vi "Shift Rev.vi"(10 "iterator":refnum<data-value>, 11 "INode in":refnum<class "INode.lvclass">) -> (3 "INode out":refnum<class "INode.lvclass">)   [LabVIEW 2023, in "d20.lvlib" / "INode.lvclass"]
uses:
  INode.lvclass
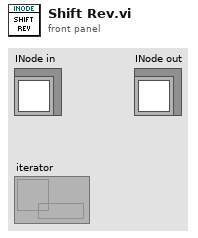
[diagram p1: front panel]
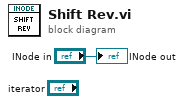
[diagram p0: block diagram]
diagram:
  "INode out" <- "INode in"
